vi "Add Channel.vi"(6 "speed (high)":i32(ring) items=["high", "low"], 8 "error in":errorcluster, 9 "direction (incoming)":i32(ring) items=["incoming", "outgoing"], 10 "hardwareChannel":i32, 11 "parameter file in":refnum<k24>) -> (0 "error out":errorcluster, 2 "new channel":refnum<k24>, 3 "parameter file out":refnum<k24>)   [LabVIEW 2020, in "AIM_429_Parameter_ni.lvlib"]
uses:
  AIM_429_Parameter_ni.lvlib
  C:/Users/Administrator/Desktop/GIT/Ballard-Arinc-429-XML-Generator/Source/Assemblies/Aim_Parameter_ni/bin/Debug/AIM_429_Parameter_ni.dll
  Assemblies/Aim_Parameter_ni/bin/Debug/AIM_429_Parameter_ni.dll
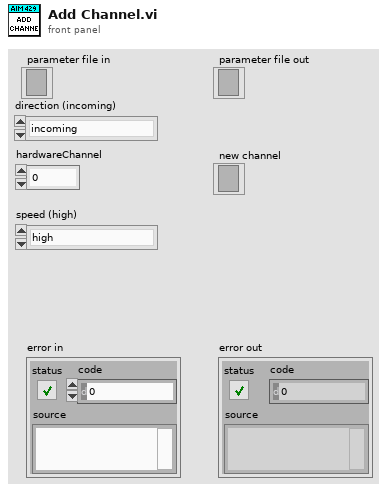
[diagram p1: front panel]
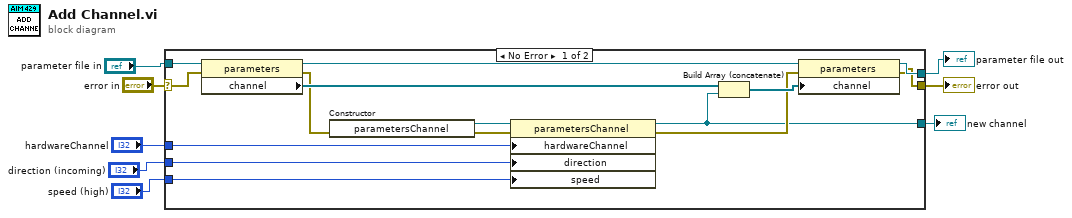
[diagram p0: block diagram]
diagram:
  n1 = case shown="No Error" "error in" {
    selector: "error in" -> [w22 w24]
    tunnel: [w18 w25] -> w8
    tunnel: [w17 w24] -> w7
    tunnel: "parameter file in" -> [w23 w25]
    tunnel: [w11 _] -> w3
    tunnel: "hardwareChannel" -> [w12 _]
    tunnel: "direction (incoming)" -> [w10 _]
    tunnel: "speed (high)" -> [w9 _]
    frame No Error {
      n2 = property class="parameters"(reference=w23, error in=w22) -> (reference out=w19:refnum<k24>, error out=w20:errorcluster, "channel"=w21:refnum<k24>[])
      n3 = constructor class="parametersChannel"(error in=w20) -> (reference out=w15:refnum<k24>, error out=w14:errorcluster)  [unwired: 2 in, 1 out]
      n4 = property class="parametersChannel"(reference=w15, error in=w14, "hardwareChannel"=w12, "direction"=w10, "speed"=w9) -> (reference out=w11:refnum<k24>, error out=w13:errorcluster)
      n5 = Build Array (concatenate)(w21, w11) -> (w16:refnum<k24>[])
      n6 = property class="parameters"(reference=w19, error in=w13, "channel"=w16) -> (reference out=w18:refnum<k24>, error out=w17:errorcluster)
    }
    frame Error {
    }
  }
  "parameter file out" <- w8
  "error out" <- w7
  "new channel" <- w3
